vi "Pársorsoló.vi"() -> ()   [LabVIEW 2014]
doc: "Pársorsoló alkalmazás.\nÖsszesorsol párokat, majd ezeket kiírja, fel olvassa és naplózza is.s\n\n-----------------------------------------------------------------------\nHasználati útmutató:\n1. Az alkalmazás mappáján belül a \"csapatok.txt\" fájlt módosítsa a csapatok aktuális felépítésének megfelelõen.\n 2. A 2 csapat tagjait láthatja ABC sorrendben a \"A csapatok tagjai\" felirat alatt.\n 3. Nyomja meg a \"Sorsolás\" gombot a véletlenszerû párosításhoz.\n 4. A kisorsolt párosítást láthatja a \"Az összesorsolt párok\" felirat alatt.\n 5. Ezt a párosítást a \"Felolvasás\" gomb lenyomásával a gép automatikusan felolvassa, teljes mondatokban. A felolvasás megismételhetõ.\n6. A párosításokat utólag is megtekintheti, az alkalmazás mappáján belül a \"Naplók\" mappában a dátum_x.txt naplófájlban (amiben az x az épp aktális napon keletkezett naplófájl sorszámát jelenti), ami tartalmazza a mentés idõpontját másodpercre pontosan, és a párok neveit.\n7. A naplófájlt a \"Naplófájl megnyitása\" gomb meg is jeleníti.\n8. Az \"Olvass el fájl megnyitása\" gombra kattintva megnyílik az \"Olvass el!\" fájl, ahol további információkat tudhat meg(ön most épp ezt olvassa).\n9. A program a \"Leállítás\" gomb megnyomására leáll.\n--------------------------------------------------------------------------------------"
uses:
  <vilib>/Utility/file.llb/Read From Spreadsheet File (string).vi
  <vilib>/Utility/file.llb/Write To Spreadsheet File (string).vi
panel:
  in  "HELP":bool
  in  "Leállítás":bool
  in  "Újra":bool
  in  "Megnyitás":bool
  out "HIBA":bool
  in  "Módosítás":bool
  in  "Felolvasás":bool
  in  "Sorsolás":bool
  out "A \"B\" csapat játékosai:":string[](array[string])
  out "Az összesorsolt párok :\nAz \"A\" csapat játékosai:":string[](array[string])
  out "A \"B\" csapat tagjai:":string[](array[string])
  out "Az \"A\" csapat tagjai:":string[](array[string])
  # "A csapatok tagjai :"
  # "Rövid leírás:"
  # "1. Az alkalmazás mappáján belül a \"csapatok.txt\" fájlt módosítsa a csapatok\n    aktuális felépítésének megfelelõen.\n2. A 2 csapat tagjait láthatja ABC sorrendben a \"A csapatok tagjai\" felirat alatt.\n3. Nyomja meg a \"Sorsolás\" gombot a véletlenszerû párosításhoz.\n4. A kisorsolt párosítást láthatja a \"Az összesorsolt párok\" felirat alatt.\n5. Ezt a párosítást a \"Felolvasás\" gomb lenyomásával a gép automatikusan\n    felolvassa, teljes mondatokban.  A felolvasás megismételhetõ.\n6. A párosításokat utólag is megtekintheti, az alkalmazás mappáján belül a \n    \"Naplók\" mappában.\n7. A naplófájlt a \"Naplófájl megnyitása\" gomb meg is jeleníti.\n8. Az \"Olvass el fájl megnyitása\" gombra kattintva megnyílik az \"Olvass el!\" fájl,\n    ahol további információkat tudhat meg.\n9. A program a \"Leállítás\" gomb megnyomására leáll."
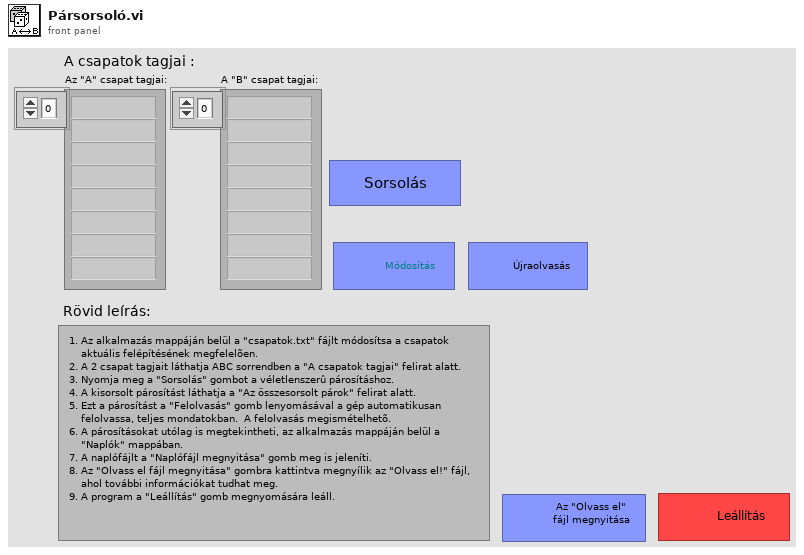
[diagram p1: front panel]
types:
  T1 = enum16{"open", "replace", "create", "open or create", "replace or create", "replace or create with confirmation"}
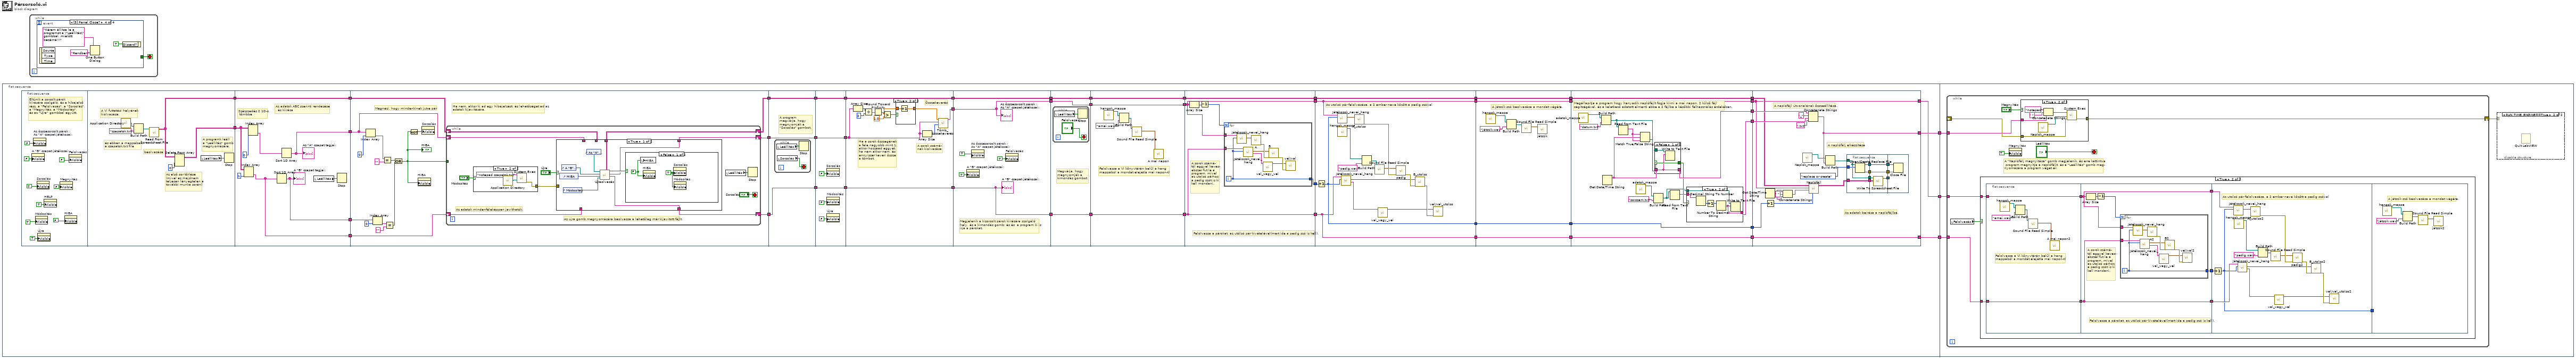
[diagram p0: block diagram]
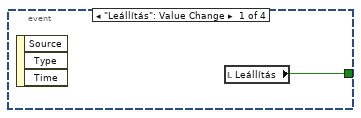
[diagram p2: hidden frame]
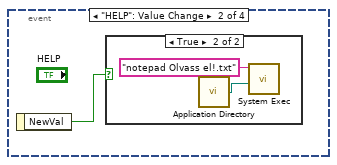
[diagram p3: hidden frame]
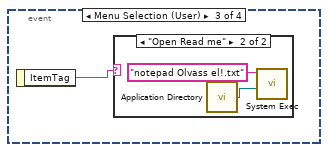
[diagram p5: hidden frame]
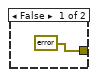
[diagram p7: hidden frame]
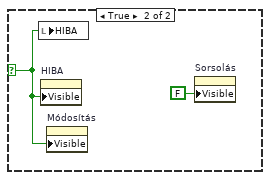
[diagram p8: hidden frame]
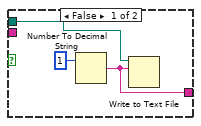
[diagram p11: hidden frame]
diagram:
  n1 = flat-sequence {
    tunnel: [w24] -> w3
    tunnel: [w8] -> w2
    tunnel: [w7] -> w1
    tunnel: w3 -> [w277]
    tunnel: w2 -> [w275]
    tunnel: w1 -> [w274]
    frame #0 {
      n2 = flat-sequence {
        tunnel: [w65] -> w51
        tunnel: [w61] -> w23
        tunnel: w51 -> [w72]
        tunnel: [w73] -> w19
        tunnel: [w69] -> w20
        tunnel: [w70] -> w18
        tunnel: w23 -> [w70]
        tunnel: [w68] -> w17
        tunnel: [w77] -> w50
        tunnel: w17 -> [w83]
        tunnel: w18 -> [w78]
        tunnel: w19 -> [w84]
        tunnel: w20 -> [w85]
        tunnel: [w80] -> w10
        tunnel: [w79] -> w9
        tunnel: [w125] -> w16
        tunnel: [w126] -> w14
        tunnel: w50 -> [w126]
        tunnel: [w124] -> w12
        tunnel: w10 -> [w125]
        tunnel: w9 -> [w124]
        tunnel: w16 -> [w134]
        tunnel: [w134] -> w15
        tunnel: w14 -> [w133]
        tunnel: [w133] -> w13
        tunnel: w12 -> [w132]
        tunnel: [w132] -> w11
        tunnel: w15 -> [w146]
        tunnel: [w136] -> w49
        tunnel: [w146] -> w48
        tunnel: [w145] -> w47
        tunnel: w13 -> [w145]
        tunnel: w11 -> [w135]
        tunnel: w49 -> [w152]
        tunnel: w48 -> [w153]
        tunnel: [w153] -> w46
        tunnel: [w152] -> w45
        tunnel: [w151] -> w44
        tunnel: w47 -> [w151]
        tunnel: [w158] -> w43
        tunnel: w46 -> [w158]
        tunnel: [w157] -> w42
        tunnel: w45 -> [w157]
        tunnel: [w156] -> w41
        tunnel: w44 -> [w156]
        tunnel: [w167] -> w40
        tunnel: w43 -> [w167]
        tunnel: w42 -> [w161]
        tunnel: [w161] -> w39
        tunnel: [w162] -> w38
        tunnel: w41 -> [w162]
        tunnel: w40 -> [w168]
        tunnel: w39 -> [w171]
        tunnel: [w171] -> w35
        tunnel: [w169] -> w36
        tunnel: [w170] -> w37
        tunnel: w38 -> [w170]
        tunnel: [w168] -> w34
        tunnel: [w186] -> w33
        tunnel: [w184] -> w32
        tunnel: [w194] -> w31
        tunnel: w37 -> [w194]
        tunnel: w36 -> [w185]
        tunnel: w35 -> [w186]
        tunnel: w34 -> [w183]
        tunnel: [w183] -> w4
        tunnel: w33 -> [w206]
        tunnel: [w206] -> w30
        tunnel: w32 -> [w200]
        tunnel: w31 -> [w202]
        tunnel: [w202] -> w29
        tunnel: [w200] -> w21
        tunnel: [w199] -> w5
        tunnel: w4 -> [w199]
        tunnel: w30 -> [w223]
        tunnel: [w223] -> w25
        tunnel: w29 -> [w222]
        tunnel: [w222] -> w26
        tunnel: [w215] -> w27
        tunnel: [w213] -> w28
        tunnel: [w208] -> w22
        tunnel: w21 -> [w208]
        tunnel: [w207] -> w6
        tunnel: w5 -> [w207]
        tunnel: w28 -> [w259]
        tunnel: w27 -> [w258]
        tunnel: w26 -> [w247]
        tunnel: w25 -> [w246]
        tunnel: [w255] -> w24
        tunnel: w22 -> [w256]
        tunnel: [w246] -> w8
        tunnel: [w245] -> w7
        tunnel: w6 -> [w245]
        frame #0 {
          # "Eltûnik a sorsolt párok\nkiírására szolgáló, és a hibajelzõ\nrész, a \"Felolvasás\", a \"Sorsolás\",\na \"Megnyitás, a \"Módosítás\",\nés az \"Újra\" gombbal együtt."
          n3 = property on="A \"B\" csapat játékosai:" class="Arr (strict)"("Visible"=FALSE) -> ()  [unwired: 2 in, 2 out]
          n4 = property on="Az összesorsolt párok :\nAz \"A\" csapat játékosai:" class="Arr (strict)"("Visible"=FALSE) -> ()  [unwired: 2 in, 2 out]
          n5 = property on="Módosítás" class="Bool (strict)"("Visible"=TRUE) -> ()  [unwired: 2 in, 2 out]
          n6 = property on="Sorsolás" class="Bool (strict)"("Visible"=TRUE) -> ()  [unwired: 2 in, 2 out]
          n7 = property on="Újra" class="Bool (strict)"("Visible"=TRUE) -> ()  [unwired: 2 in, 2 out]
          n8 = property on="HELP" class="Bool (strict)"("Visible"=TRUE) -> ()  [unwired: 2 in, 2 out]
          n9 = property on="Megnyitás" class="Bool (strict)"("Visible"=FALSE) -> ()  [unwired: 2 in, 2 out]
          n10 = property on="HIBA" class="Bool (strict)"("Visible"=FALSE) -> ()  [unwired: 2 in, 2 out]
          n11 = property on="Felolvasás" class="Bool (strict)"("Visible"=FALSE) -> ()  [unwired: 2 in, 2 out]
        }
        frame #1 {
          # "A programk leáll\na \"Leállítás\" gomb\nmegnyomására."
          # "Az elsõ sor törlése\n(mivel ez majdnem\nteljesen lényegtelen a \ntovábbi munka során)"
          # "beolvasása"
          # "és ebben a mappában\na csapatok.txt file"
          # "A Vi futtatási helyének\nkiolvasása,"
          n12 = call <vilib>:"Application Directory.vi"() -> ("Application Directory"=w64:path)
          n13 = Build Path(base path=w64, name or relative path="csapatok.txt") -> (appended path=w63:path)
          n14 = call-poly <vilib>:"Read From Spreadsheet File.vi"("file path (dialog if empty)"=w63) -> ("all rows"=w61:string[][])  [unwired: 6 in, 4 out]
          n15 = Delete From Array(array=w61, index (row)=0) -> (array with subset deleted=w65:string[][])  [unwired: 2 in, 1 out]
          n16 = local read "Leállítás"() -> (w62:bool)
          n17 = Stop(stop? (T)=w62) -> ()
        }
        frame #2 {
          # "Szézszedés 2 1D-s\n tömbbe"
          # "Az adatok ABC szerinti rendezése\n, és kiírása"
          n18 = Index Array(array=w72, index (col)=1 ("disabled index (col)")) -> (element=w68:string[])  [unwired: 1 in]
          n19 = Index Array(array=w72, index (col)=0 ("disabled index (col)")) -> (element=w74:string[])  [unwired: 1 in]
          n20 = Sort 1D Array(array=w68) -> (sorted array=w69:string[])
          "A \"B\" csapat tagjai:" <- w69
          n21 = Sort 1D Array(array=w74) -> (sorted array=w73:string[])
          "Az \"A\" csapat tagjai:" <- w73
          n22 = local read "Leállítás"() -> (w71:bool)
          n23 = Stop(stop? (T)=w71) -> ()
        }
        frame #3 {
          # "Ha nem, akkor ki ad egy hibajelzést, és lehetõséget ad az\nadatok kijavítására."
          # "Megnézi, hogy mindenkinek jut-e pár"
          n24 = Index Array(array=w84, index=0) -> (element=w92:string)
          n25 = Index Array(array=w85, index=0) -> (element=w91:string)
          n26 = Equal?(x=w92, y="") -> (x = y?=w88:bool)
          n27 = Equal?(x=w91, y="") -> (x = y?=w87:bool)
          n28 = Or(x=w88, y=w87) -> (x .or. y?=w81:bool)
          "HIBA" <- w81
          n29 = Not(x=w81) -> (.not. x?=w82:bool)
          n30 = property on="HIBA" class="Bool (strict)"("Visible"=w81) -> ()  [unwired: 2 in, 2 out]
          n31 = property on="Sorsolás" class="Bool (strict)"("Visible"=w82) -> ()  [unwired: 2 in, 2 out]
          n32 = while {
            tunnel: w81 -> [_]
            shift-right: [w96] -> w79
            shift-left: w84 -> [w102]
            shift-right: [w97] -> w80
            shift-left: w83 -> [w103]
            shift-right: [w95] -> w77
            shift-left: w78 -> [w94]
            stop <- "Sorsolás" stop-if-true
            # "Az adatok mindenféleképpen javíthatók."
            # "Az újra gomb megnyomására beolvassa a lehetõleg már kijavított fájlt."
            n33 = case shown="True" "Módosítás" {
              tunnel: [errorcluster {"status"=FALSE, "code"=0, "source"=""} ("error in (no error)") w106] -> w100
              frame False {
              }
              frame True {
                n34 = call <vilib>:"Application Directory.vi"() -> ("Application Directory"=w108:path)
                n35 = call <vilib>:"System Exec.vi"("working directory"=w108, "command line"="notepad csapatok.txt") -> ("error out"=w106:errorcluster)  [unwired: 6 in, 3 out]
              }
            }
            n36 = case shown="True" "Újra" {
              tunnel: [w110 w122] -> w96
              tunnel: [w111 w123] -> w97
              tunnel: w103 -> [_ w123]
              tunnel: w102 -> [_ w122]
              tunnel: w100 -> [_ _]
              tunnel: [w109 w121] -> w95
              tunnel: w94 -> [_ w121]
              frame True {
                n37 = control-ref of="HIBA"() -> (w113:refnum<vi>)
                n38 = control-ref of="A \"B\" csapat tagjai:"() -> (w112:refnum<vi>)
                n39 = control-ref of="Módosítás"() -> (w114:refnum<vi>)
                n40 = control-ref of="Az \"A\" csapat tagjai:"() -> (w115:refnum<vi>)
                n41 = call "Újraolvasás.vi"("Módosítás láthatóság"=w114, "HIBA láthatóság"=w113, "B csapat tagjai"=w112, "A csapat tagjai"=w115) -> ("B csapat tagjai kimenet"=w111:string[], "A csapat tagjai kimenet"=w110:string[], "Mindenkinek van párja?"=w116:bool, "Original file"=w109:string[][])  [unwired: 4 in]
                n42 = case shown="False" w116 {
                  selector: w116 -> [_ w119]
                  frame False {
                    w118 = FALSE ("Visible")
                    w117 = TRUE ("Visible")
                    n43 = local write "HIBA"(w118) -> ()
                    n44 = property on="HIBA" class="Bool (strict)"("Visible"=w118) -> ()  [unwired: 2 in, 2 out]
                    n45 = property on="Sorsolás" class="Bool (strict)"("Visible"=w117) -> ()  [unwired: 2 in, 2 out]
                    n46 = property on="Módosítás" class="Bool (strict)"("Visible"=w117) -> ()  [unwired: 2 in, 2 out]
                  }
                  frame True {
                    n47 = local write "HIBA"(w119) -> ()
                    n48 = property on="HIBA" class="Bool (strict)"("Visible"=w119) -> ()  [unwired: 2 in, 2 out]
                    n49 = property on="Módosítás" class="Bool (strict)"("Visible"=w119) -> ()  [unwired: 2 in, 2 out]
                    n50 = property on="Sorsolás" class="Bool (strict)"("Visible"=FALSE) -> ()  [unwired: 2 in, 2 out]
                  }
                }
              }
              frame False {
              }
            }
            n51 = local read "Leállítás"() -> (w98:bool)
            n52 = Stop(stop? (T)=w98) -> ()
          }
        }
        frame #4 {
          # "A program \nmegvárja, hogy\nmegnyomják a\n\"Sorsolás\" gombot."
          n53 = while {
            stop <- w127 stop-if-true
            n54 = local read "Leállítás"() -> (w128:bool)
            n55 = local read "Sorsolás"() -> (w127:bool)
            n56 = Stop(stop? (T)=w128) -> ()
          }
        }
        frame #5 {
          n57 = property on="Sorsolás" class="Bool (strict)"("Visible"=FALSE) -> ()  [unwired: 2 in, 2 out]
          n58 = property on="Módosítás" class="Bool (strict)"("Visible"=FALSE) -> ()  [unwired: 2 in, 2 out]
          n59 = property on="Újra" class="Bool (strict)"("Visible"=FALSE) -> ()  [unwired: 2 in, 2 out]
        }
        frame #6 {
          # "Ha a sorok összegének\na fele nagyobb mint 1,\nakkor hozzáad eggyet,\nha nem akkor nem, és\nennyiszer keveri össze\na tömbot."
          # "A sorok számá-\nnak kiolvasása"
          # "Összekeverés"
          n60 = Array Size(array=w135) -> (size(s)=w143:i32)
          n61 = Divide(x=w143, y=2) -> (x/y=w141:dbl)
          n62 = Round Toward +Infinity(x=w141) -> (ceil(x): smallest int >= x=w138:dbl)
          n63 = Greater?(x=w138, y=1.0) -> (0:w139:bool)
          n64 = case shown="True" w139 {
            tunnel: w138 -> [w147 w149]
            tunnel: [w147 w148] -> w137
            frame False {
            }
            frame True {
              n65 = Increment(x=w149) -> (x+1=w148:dbl)
            }
          }
          n66 = Array Size(array=w135) -> (size(s)=w144:i32)
          n67 = call "Tömb_összekeverés.vi"("Sorok száma"=w144, "Keverendõ tömb(1D)"=w135, "Sorsolás ism. száma"=w137) -> ("Összekevert tömb"=w136:string[])  [unwired: 8 in]
        }
        frame #7 {
          # "Megjelenik a kisorsolt párok kiírására szolgáló\nhely, és a kimondás gomb; és és  a program ki is\nírja a párokat."
          n68 = property on="A \"B\" csapat játékosai:" class="Arr (strict)"("Visible"=TRUE) -> ()  [unwired: 2 in, 2 out]
          n69 = property on="Az összesorsolt párok :\nAz \"A\" csapat játékosai:" class="Arr (strict)"("Visible"=TRUE) -> ()  [unwired: 2 in, 2 out]
          n70 = property on="Felolvasás" class="Bool (strict)"("Visible"=TRUE) -> ()  [unwired: 2 in, 2 out]
          "Az összesorsolt párok :\nAz \"A\" csapat játékosai:" <- w152
          "A \"B\" csapat játékosai:" <- w153
        }
        frame #8 {
          # "Megvárja, hogy\nmegnyomják a\nkimondás gombot"
          n71 = while {
            stop <- "Felolvasás" stop-if-true
            n72 = local read "Leállítás"() -> (w159:bool)
            n73 = Stop(stop? (T)=w159) -> ()
          }
        }
        frame #9 {
          # "Felolvassa a Vi könyvtárán belül a hang\nmappából a mondat elejét(a mai napon-t)"
          n74 = call "hangok_mappa.vi"() -> ("*\\hang mapppa"=w163:path)  [unwired: 11 in]
          n75 = Build Path(base path=w163, name or relative path="amai.wav") -> (appended path=w165:path)
          n76 = call <vilib>:"Sound File Read Simple.vi"("path"=w165) -> ("data"=w166:waveform(dbl)[])  [unwired: 7 in, 3 out]
          n77 = call "A mai napon"("Data"=w166) -> ()  [unwired: 18 in, 1 out]
        }
        frame #10 {
          # "A sorok számá-\ntól eggyel keves-\nebszer fut le a\nprogram, mivel\naz utolsó párhoz\na pedig szót is ki\nkell mondani."
          # "Felolvassa a párokat, az utólsó pár kivételével(mert ide a pedig szó is kell)."
          n78 = Array Size(array=w171) -> (size(s)=w173:i32)
          n79 = Decrement(x=w173) -> (x-1=w172:i32)
          n80 = for {
            N: w172 -> [_]
            tunnel: w171 -> [w182]
            tunnel: w168 -> [w175]
            tunnel: [w174] -> w169
            i -> [w174]
            n81 = call "Játékosok_nevei_hang.vi"("Index"=w174, "Játékosok(1D tömb)"=w182) -> ("Becenév hang"=w181:waveform(dbl)[])  [unwired: 8 in, 1 out]
            n82 = call "Játékosok_nevei_hang.vi"("Index"=w174, "Játékosok(1D tömb)"=w175) -> ("Becenév"=w177:string, "Becenév hang"=w176:waveform(dbl)[])  [unwired: 8 in]
            n83 = call "A"("Data"=w181) -> ("error out"=w180:errorcluster)  [unwired: 18 in]
            n84 = call "val_vagy_vel.vi"("Becenév"=w177) -> ("-val/vel rag"=w178:waveform(dbl)[])  [unwired: 10 in]
            n85 = call "B"("Data"=w176, "error in"=w180) -> ("error out"=w179:errorcluster)  [unwired: 17 in]
            n86 = call "vel/val"("Data"=w178, "error in"=w179) -> ()  [unwired: 17 in, 1 out]
          }
        }
        frame #11 {
          # "Az utolsó pár felolvasása, a 2 ember neve között a pedig szóval"
          n87 = Increment(x=w185) -> (x+1=w184:i32)
          n88 = call "Játékosok_nevei_hang.vi"("Index"=w184, "Játékosok(1D tömb)"=w186) -> ("Becenév hang"=w193:waveform(dbl)[])  [unwired: 8 in, 1 out]
          n89 = call "hangok_mappa.vi"() -> ("*\\hang mapppa"=w192:path)  [unwired: 11 in]
          n90 = call "Játékosok_nevei_hang.vi"("Index"=w184, "Játékosok(1D tömb)"=w183) -> ("Becenév"=w189:string, "Becenév hang"=w190:waveform(dbl)[])  [unwired: 8 in]
          n91 = call "A_utolso"("Data"=w193) -> ("error out"=w197:errorcluster)  [unwired: 18 in]
          n92 = Build Path(base path=w192, name or relative path="pedig.wav") -> (appended path=w196:path)
          n93 = call <vilib>:"Sound File Read Simple.vi"("path"=w196) -> ("data"=w195:waveform(dbl)[])  [unwired: 7 in, 3 out]
          n94 = call "val_vagy_vel.vi"("Becenév"=w189) -> ("-val/vel rag"=w187:waveform(dbl)[])  [unwired: 10 in]
          n95 = call "pedig"("Data"=w195, "error in"=w197) -> ("error out"=w191:errorcluster)  [unwired: 17 in]
          n96 = call "B_utolso"("Data"=w190, "error in"=w191) -> ("error out"=w188:errorcluster)  [unwired: 17 in]
          n97 = call "vel/val_utolso"("Data"=w187, "error in"=w188) -> ()  [unwired: 17 in, 1 out]
        }
        frame #12 {
          # "A játszik szó beolvasása a mondat végére."
          n98 = call "hangok_mappa.vi"() -> ("*\\hang mapppa"=w201:path)  [unwired: 11 in]
          n99 = Build Path(base path=w201, name or relative path="játszik.wav") -> (appended path=w204:path)
          n100 = call <vilib>:"Sound File Read Simple.vi"("path"=w204) -> ("data"=w205:waveform(dbl)[])  [unwired: 7 in, 3 out]
          n101 = call "játszik"("Data"=w205) -> ()  [unwired: 18 in, 1 out]
        }
        frame #13 {
          # "Megállapítja a program hogy hanyadik naplófájlt fogja kiírni a mai napon, 2 külsõ fájl\nsegítségével, és a keletkezõ adatott elmenti ebbe a 2 fájlba a késõbbi felhasználás érdekében."
          n102 = call "adatok_mappa.vi"() -> ("*\\adatok mappa útvonala"=w220:path)  [unwired: 11 in]
          n103 = Build Path(base path=w220, name or relative path="datum.txt") -> (appended path=w212:path)
          n104 = Get Date/Time String() -> (date string=w219:string)  [unwired: 3 in, 1 out]
          n105 = Read from Text File(file (use dialog)=w212) -> (text=w209:string)  [unwired: 3 in, 3 out]
          n106 = call "adatok_mappa.vi"() -> ("*\\adatok mappa útvonala"=w210:path)  [unwired: 11 in]
          n107 = Match True/False String(2:w209, 3:w219, 4:w209) -> (0:w218:bool)  [unwired: 1 out]
          n108 = Build Path(base path=w210, name or relative path="sorszam.txt") -> (appended path=w211:path)
          n109 = case shown="False" w218 {
            selector: w218 -> [w234 w235]
            tunnel: w219 -> [w233 w236]
            tunnel: [w233 w236] -> w215
            tunnel: [w234 w235] -> w214
            tunnel: w212 -> [w232 _]
            frame False {
              n110 = Write to Text File(file (use dialog)=w232, text=w233) -> ()  [unwired: 2 in, 3 out]
            }
            frame True {
            }
          }
          n111 = Read from Text File(file (use dialog)=w211) -> (text=w216:string)  [unwired: 3 in, 3 out]
          n112 = case shown="True" w214 {
            tunnel: w216 -> [_ w229]
            tunnel: [w225 w228] -> w213
            tunnel: w211 -> [w224 w227]
            frame False {
              n113 = Number To Decimal String(number=1) -> (decimal integer string=w225:string)  [unwired: 1 in]
              n114 = Write to Text File(file (use dialog)=w224, text=w225) -> ()  [unwired: 2 in, 3 out]
            }
            frame True {
              n115 = Decimal String To Number(string=w229) -> (number=w230:i32)  [unwired: 2 in, 1 out]
              n116 = Increment(x=w230) -> (x+1=w231:i32)
              n117 = Number To Decimal String(number=w231) -> (decimal integer string=w228:string)  [unwired: 1 in]
              n118 = Write to Text File(file (use dialog)=w227, text=w228) -> ()  [unwired: 2 in, 3 out]
            }
          }
        }
        frame #14 {
          # "Az adatok beírása a naplófájlba."
          # "A naplófálj elkészítése"
          # "A naplófájl útvonalának összeállítása."
          n119 = Get Date/Time String() -> (date string=w249:string, time string=w250:string)  [unwired: 3 in]
          n120 = Increment(x=w256) -> (x+1=w253:i32)
          n121 = Concatenate Strings(w249, " " ("string"), w250) -> (w248:string)
          n122 = call "Naplók_mappa.vi"() -> ("*\\Naplók útvonala"=w260:path)  [unwired: 11 in]
          n123 = Concatenate Strings(w258, "_" ("string"), w259, ".txt" ("name or relative path")) -> (w255:string)
          n124 = call "Naplófájl.vi"("Index"=w253, "Dátum(string)"=w248, "Összekevert tömb"=w246, "Eredeti tömb"=w247) -> ("Kész naplófájl(2D Tömb)"=w242:string[][])  [unwired: 7 in]
          n125 = Build Path(base path=w260, name or relative path=w255) -> (appended path=w252:path)
          n126 = flat-sequence {
            tunnel: T1."replace or create" ("operation (0:open)") -> [w266]
            tunnel: w252 -> [w262]
            tunnel: [w265] -> w244
            tunnel: [w264] -> w243
            tunnel: w242 -> [w263]
            tunnel: [w263] -> w241
            tunnel: [w262] -> w240
            tunnel: w244 -> [w271]
            tunnel: w243 -> [w270]
            tunnel: w241 -> [w269]
            tunnel: w240 -> [w268]
            tunnel: [w271] -> w239
            tunnel: [w270] -> w238
            tunnel: [w267] -> w237
            tunnel: w239 -> [w273]
            tunnel: w238 -> [w272]
            tunnel: w237 -> [_]
            frame #0 {
              n127 = Open/Create/Replace File(file path (use dialog)=w262, operation (0:open)=w266) -> (refnum out=w264:refnum<file>, error out=w265:errorcluster)  [unwired: 4 in, 1 out]
            }
            frame #1 {
              n128 = call-poly <vilib>:"Write To Spreadsheet File.vi"("2D data"=w269, "file path (dialog if empty)"=w268) -> ("new file path (Not A Path if cancelled)"=w267:path)  [unwired: 6 in]
            }
            frame #2 {
              n129 = Close File(refnum=w272, error in=w273) -> ()  [unwired: 2 out]
            }
          }
        }
      }
    }
    frame #1 {
      n130 = while {
        tunnel: w277 -> [w284]
        shift-right: [w282] -> w276
        shift-left: _ -> [w281]
        tunnel: w275 -> [w280]
        tunnel: w274 -> [w279]
        stop <- "Leállítás" stop-if-true
        # "A \"Naplófálj megnyitása\" gomb megjelenik, és erre kattintva\n program megnyitja a naplófáljt, és a \"Leállítás\" gomb meg-\nnyomására a program véget ér."
        n131 = local read "Felolvasás"() -> (w278:bool)
        n132 = case shown="True" w278 {
          tunnel: w280 -> [_ w288]
          tunnel: w279 -> [_ w287]
          frame False {
          }
          frame True {
            n133 = flat-sequence {
              tunnel: [w295] -> w294
              tunnel: [w296] -> w293
              tunnel: w288 -> [w296]
              tunnel: w287 -> [w295]
              tunnel: w294 -> [w301]
              tunnel: w293 -> [w303]
              tunnel: [w303] -> w291
              tunnel: [w302] -> w292
              tunnel: [w301] -> w290
              tunnel: [w315] -> w289
              tunnel: w292 -> [w316]
              tunnel: w291 -> [w318]
              tunnel: w290 -> [w317]
              tunnel: w289 -> [_]
              frame #0 {
                # "Felolvassa a Vi könyvtárán belül a hang\nmappából a mondat elejét(a mai napon-t)"
                n134 = call "hangok_mappa.vi"() -> ("*\\hang mapppa"=w297:path)  [unwired: 11 in]
                n135 = Build Path(base path=w297, name or relative path="amai.wav") -> (appended path=w299:path)
                n136 = call <vilib>:"Sound File Read Simple.vi"("path"=w299) -> ("data"=w300:waveform(dbl)[])  [unwired: 7 in, 3 out]
                n137 = call "A mai napon2"("Data"=w300) -> ()  [unwired: 18 in, 1 out]
              }
              frame #1 {
                # "A sorok számá-\ntól eggyel keves-\nebszer fut le a\nprogram, mivel\naz utolsó párhoz\na pedig szót is ki\nkell mondani."
                # "Felolvassa a párokat, az utólsó pár kivételével(mert ide a pedig szó is kell)."
                n138 = Array Size(array=w303) -> (size(s)=w305:i32)
                n139 = Decrement(x=w305) -> (x-1=w304:i32)
                n140 = for {
                  N: w304 -> [_]
                  tunnel: w303 -> [w314]
                  tunnel: w301 -> [w307]
                  tunnel: [w306] -> w302
                  i -> [w306]
                  n141 = call "Játékosok_nevei_hang.vi"("Index"=w306, "Játékosok(1D tömb)"=w314) -> ("Becenév hang"=w313:waveform(dbl)[])  [unwired: 8 in, 1 out]
                  n142 = call "Játékosok_nevei_hang.vi"("Index"=w306, "Játékosok(1D tömb)"=w307) -> ("Becenév"=w309:string, "Becenév hang"=w308:waveform(dbl)[])  [unwired: 8 in]
                  n143 = call "A2"("Data"=w313) -> ("error out"=w312:errorcluster)  [unwired: 18 in]
                  n144 = call "val_vagy_vel.vi"("Becenév"=w309) -> ("-val/vel rag"=w310:waveform(dbl)[])  [unwired: 10 in]
                  n145 = call "B2"("Data"=w308, "error in"=w312) -> ("error out"=w311:errorcluster)  [unwired: 17 in]
                  n146 = call "vel/val2"("Data"=w310, "error in"=w311) -> ()  [unwired: 17 in, 1 out]
                }
              }
              frame #2 {
                # "Az utolsó pár felolvasása, a 2 ember neve között a pedig szóval"
                n147 = Increment(x=w316) -> (x+1=w315:i32)
                n148 = call "Játékosok_nevei_hang.vi"("Index"=w315, "Játékosok(1D tömb)"=w318) -> ("Becenév hang"=w325:waveform(dbl)[])  [unwired: 8 in, 1 out]
                n149 = call "hangok_mappa.vi"() -> ("*\\hang mapppa"=w324:path)  [unwired: 11 in]
                n150 = call "Játékosok_nevei_hang.vi"("Index"=w315, "Játékosok(1D tömb)"=w317) -> ("Becenév"=w321:string, "Becenév hang"=w322:waveform(dbl)[])  [unwired: 8 in]
                n151 = call "A_utolso2"("Data"=w325) -> ("error out"=w328:errorcluster)  [unwired: 18 in]
                n152 = Build Path(base path=w324, name or relative path="pedig.wav") -> (appended path=w327:path)
                n153 = call <vilib>:"Sound File Read Simple.vi"("path"=w327) -> ("data"=w326:waveform(dbl)[])  [unwired: 7 in, 3 out]
                n154 = call "val_vagy_vel.vi"("Becenév"=w321) -> ("-val/vel rag"=w319:waveform(dbl)[])  [unwired: 10 in]
                n155 = call "pedig2"("Data"=w326, "error in"=w328) -> ("error out"=w323:errorcluster)  [unwired: 17 in]
                n156 = call "B_utolso2"("Data"=w322, "error in"=w323) -> ("error out"=w320:errorcluster)  [unwired: 17 in]
                n157 = call "vel/val_utolso2"("Data"=w319, "error in"=w320) -> ()  [unwired: 17 in, 1 out]
              }
              frame #3 {
                # "A játszik szó beolvasása a mondat végére."
                n158 = call "hangok_mappa.vi"() -> ("*\\hang mapppa"=w330:path)  [unwired: 11 in]
                n159 = Build Path(base path=w330, name or relative path="játszik.wav") -> (appended path=w332:path)
                n160 = call <vilib>:"Sound File Read Simple.vi"("path"=w332) -> ("data"=w333:waveform(dbl)[])  [unwired: 7 in, 3 out]
                n161 = call "játszik2"("Data"=w333) -> ()  [unwired: 18 in, 1 out]
              }
            }
          }
        }
        n162 = property on="Megnyitás" class="Bool (strict)"("Visible"=TRUE) -> ()  [unwired: 2 in, 2 out]
        n163 = case shown="True" "Megnyitás" {
          tunnel: w284 -> [_ w338]
          tunnel: [w334 w336] -> w282
          tunnel: w281 -> [w334 w335]
          frame False {
          }
          frame True {
            n164 = call "Naplók_mappa.vi"() -> ("*\\Naplók útvonala"=w341:path)  [unwired: 11 in]
            n165 = Concatenate Strings("notepad" ("string"), " " ("string"), w338) -> (w337:string)
            n166 = call <vilib>:"System Exec.vi"("error in (no error)"=w335, "working directory"=w341, "command line"=w337) -> ("error out"=w336:errorcluster)  [unwired: 5 in, 3 out]
          }
        }
      }
      n167 = disable-structure shown="RUN_TIME_ENGINE==True" {
        disable-tunnel: w276 -> [_ _]
        frame condition #0 (active) {
        }
        frame condition #1 {
          n168 = Quit LabVIEW() -> ()  [unwired: 1 in]
        }
      }
    }
  }
  n169 = while {
    stop <- w342 stop-if-true
    n170 = event shown="[3] Panel Close?" {
      selector: _ -> [_ _ _ _]
      dyn-events: _ -> [_ _ _ _]
      timeout: _ -> [_ _ _ _]
      tunnel: [w343 _ _ _] -> w342
      event "Leállítás": Value Change {
        n171 = event-data() -> ()  [unwired: 1 in, 3 out]
        n172 = local read "Leállítás"() -> (w343:bool)
      }
      event "HELP": Value Change {
        n173 = event-data() -> ("NewVal"=w344:bool)  [unwired: 1 in]
        n174 = case shown="True" w344 {
          frame False {
          }
          frame True {
            n175 = call <vilib>:"Application Directory.vi"() -> ("Application Directory"=w345:path)
            n176 = call <vilib>:"System Exec.vi"("working directory"=w345, "command line"="notepad Olvass el!.txt") -> ()  [unwired: 6 in, 4 out]
          }
        }
      }
      event Menu Selection (User) {
        n177 = event-data() -> ("ItemTag"=w347:string)  [unwired: 1 in]
        n178 = case shown="\"Open Read me\"" w347 {
          frame Default {
          }
          frame "Open Read me" {
            n179 = call <vilib>:"Application Directory.vi"() -> ("Application Directory"=w348:path)
            n180 = call <vilib>:"System Exec.vi"("working directory"=w348, "command line"="notepad Olvass el!.txt") -> ()  [unwired: 6 in, 4 out]
          }
        }
      }
      event Panel Close? {
        n181 = event-data() -> ()  [unwired: 1 in, 3 out]
        n182 = One Button Dialog(message="Kérem állítsa le a programot a \"Leállítás\" gombbal, mielõtt bezárná!!!", button name ("OK")="Rendben") -> ()  [unwired: 1 out]
        n183 = event-data("Discard?"=TRUE) -> ()  [unwired: 1 in, 1 out]
      }
    }
  }
